vi "Hold to Roof_1 port_Save Sweep Data to csv.vi"(0 "Test Information":T2={"Exp Name"="Cold Switching", "Lot"="0233A", "Wafer"="15", "Die Type"="L22", "Die X "="6", "Die Y"="8", "Exp"="1", "Die X_Y"="8"}, 1 "Filepath":path, 2 "Selected Exp Settings":T5={"Floor_Sweep_Stop_V"=36.0, "Resistance Threshold"=1.0, "Floor_Sweep_Start_V"=36.0, "Floor_Sweep_Step_V"=1.0, "Roof_Sweep_Stop_V"=36.0, "Roof_Sweep_Start_V"=36.0, "Roof_Sweep_Step_V"=1.0, "Experiment Name"="", "Meas_Type"=[0, 2, 4]}, 4 "Meas Type":string="QuickView_", 5 "Date Cluster":T3, 7 "Time":dbl[](array[numeric]), 9 "ks5080A_Meaurements":T4, 12 "PreTest Capacitance":dbl[](array[numeric]), 14 "PostTest Capacitance":dbl[](array[numeric])) -> ()   [LabVIEW 2013]
uses:
  Controls/Date Control.ctl
  Controls/Test Information.ctl
  Controls/ks5080A_Measurements.ctl
  Controls/Individual User Inputs_MultiTest.ctl
  Controls/Test Selection.ctl
  <vilib>/Utility/file.llb/Write To Spreadsheet File (string).vi
panel:
  in  "Tab Control":T1(tab)
  # "Calculation Settings"
  # "Test Settings"
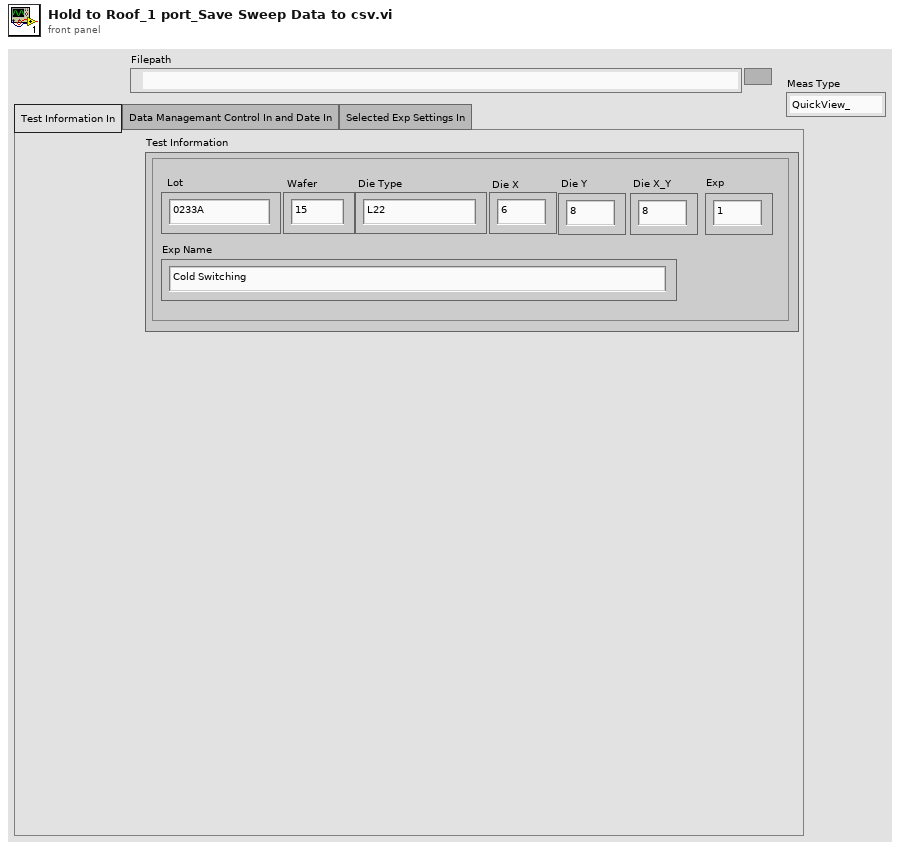
[diagram p1: front panel]
types:
  T1 = enum32{"Test Information In", "Data Managemant Control In and Date In", "Selected Exp Settings In"}
  T2 = typedef "Test Information.ctl" = cluster{"Exp Name":string, "Lot":string, "Wafer":string, "Die Type":string, "Die X ":string, "Die Y":string, "Exp":string, "Die X_Y":string}
  T3 = typedef "Date Control.ctl" = cluster{"Date":string, "Start Time":string, "Stop Time":string}
  T4 = typedef "ks5080A_Measurements.ctl" = cluster{"Bias_Sweep_Setting":dbl[], "Bias_voltage measurements":dbl[], "Bias_current measurements":dbl[], "P1_Capacitance":dbl[], "P2_Capacitance":dbl[], "DMM_Measurement_V":dbl[], "Contact_Source Current measurements":dbl[], "Contact_Sink Current measurements":dbl[], "Calculated_Resistance":dbl[], "P3_Capacitance":dbl[], "Port 1_S_parm":string[], "Port 2_S_parm":string[], "Port 3_S_parm":string[]}
  T5 = typedef "Individual User Inputs_MultiTest.ctl" = cluster{"Floor_Sweep_Stop_V":dbl, "Resistance Threshold":dbl, "Floor_Sweep_Start_V":dbl, "Floor_Sweep_Step_V":dbl, "Roof_Sweep_Stop_V":dbl, "Roof_Sweep_Start_V":dbl, "Roof_Sweep_Step_V":dbl, "Experiment Name":string, "Meas_Type":T6}
  T6 = typedef "Test Selection.ctl" = i32[]
  T7 = enum16{"open", "replace", "create", "open or create", "replace or create", "replace or create with confirmation"}
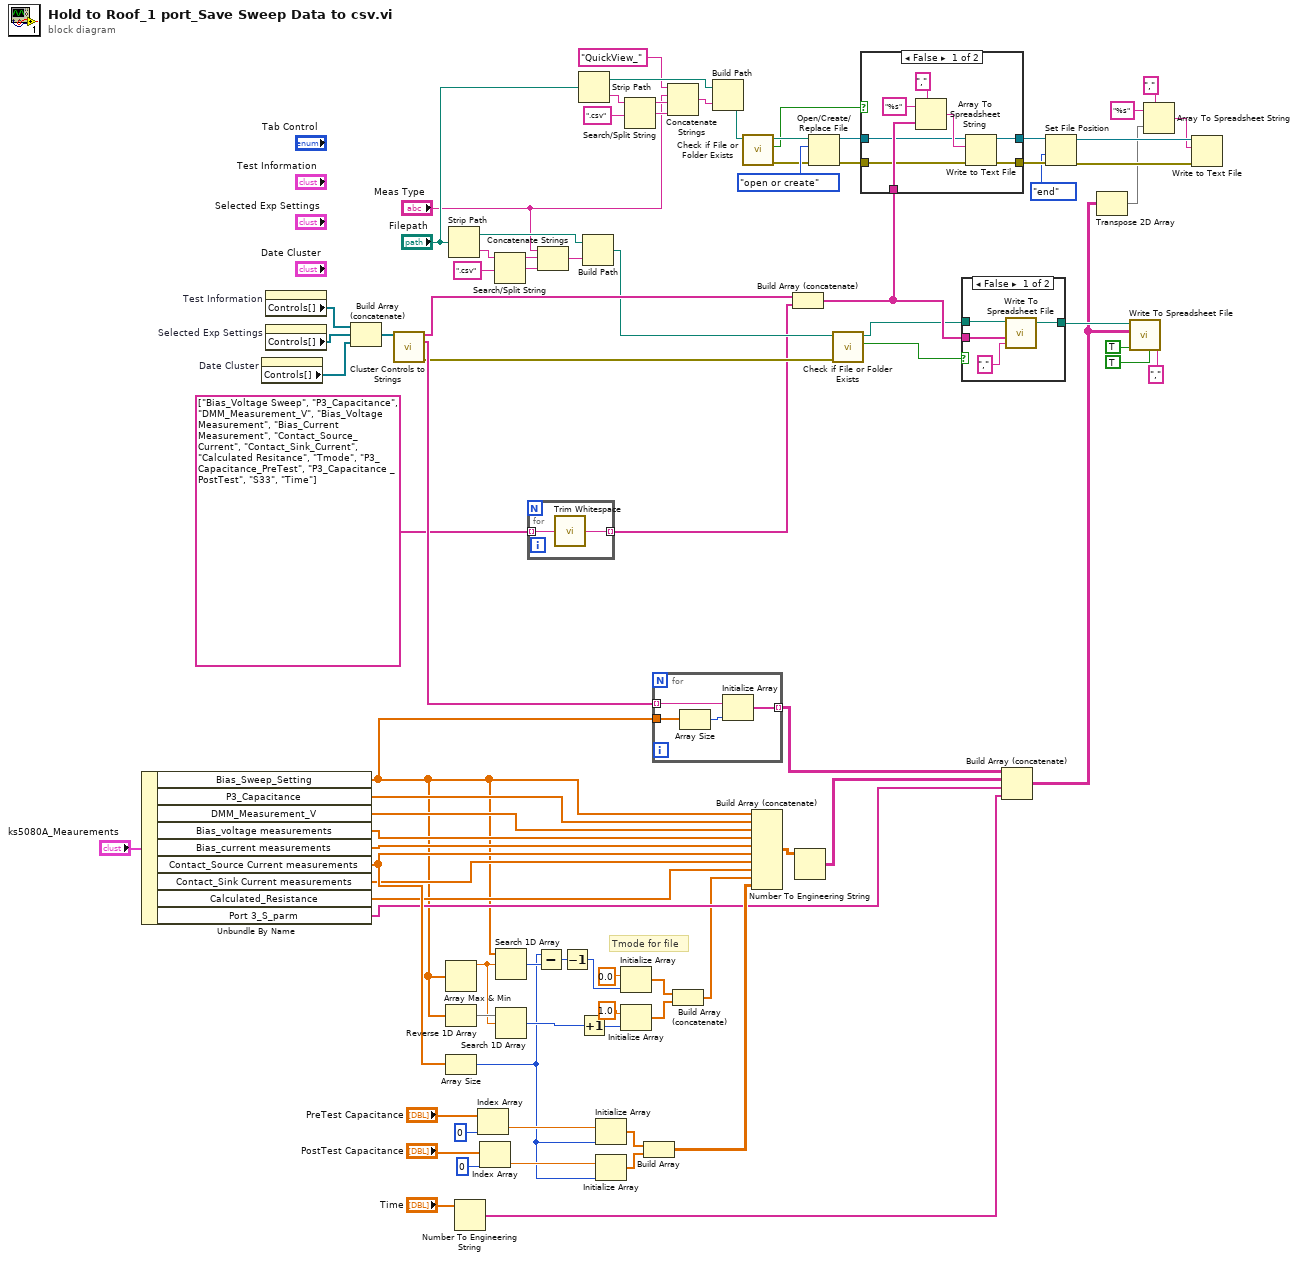
[diagram p0: block diagram]
diagram:
  # "Tmode for file"
  n1 = Unbundle By Name("ks5080A_Meaurements") -> ("Bias_Sweep_Setting"=w12:dbl[], "P3_Capacitance"=w83:dbl[], "DMM_Measurement_V"=w82:dbl[], "Bias_voltage measurements"=w81:dbl[], "Bias_current measurements"=w80:dbl[], "Contact_Source Current measurements"=w79:dbl[], "Contact_Sink Current measurements"=w48:dbl[], "Calculated_Resistance"=w47:dbl[], "Port 3_S_parm"=w30:string[])
  n2 = property on="Date Cluster" class="Clust (strict)"() -> ("Controls[]"=w1:refnum<vi>[])  [unwired: 2 in, 2 out]
  n3 = property on="Test Information" class="Clust (strict)"() -> ("Controls[]"=w86:refnum<vi>[])  [unwired: 2 in, 2 out]
  n4 = property on="Selected Exp Settings" class="Clust (strict)"() -> ("Controls[]"=w10:refnum<vi>[])  [unwired: 2 in, 2 out]
  n5 = Build Array (concatenate)(w86, w10, w1) -> (w85:refnum<vi>[])
  n6 = call "Cluster Controls to Strings.vi"("Controls[]"=w85) -> ("Control Labels"=w71:string[], "Control Values"=w84:string[], "Error Out"=w70:errorcluster)  [unwired: 12 in]
  n7 = Array Max & Min(array=w12) -> (max value=w19:dbl)  [unwired: 3 out]
  n8 = Reverse 1D Array(array=w12) -> (reversed array=w20:dbl[])
  n9 = Array Size(array=w79) -> (size(s)=w13:i32)
  n10 = Strip Path(path="Filepath") -> (stripped path=w33:path, name=w36:string)
  n11 = Number To Engineering String(4:"Time") -> (0:w8:string[])  [unwired: 3 in]
  n12 = Index Array(array="PreTest Capacitance", index=0) -> (element=w44:dbl)
  n13 = Index Array(array="PostTest Capacitance", index=0) -> (element=w43:dbl)
  n14 = Search/Split String(string=w36, search string/char (-)=".csv" ("search string")) -> (substring before match=w31:string, match + rest of string=w34:string)  [unwired: 1 in, 1 out]
  n15 = Search 1D Array(1D array=w12, element=w19) -> (index of element=w18:i32)  [unwired: 1 in]
  n16 = Search 1D Array(1D array=w20, element=w19) -> (index of element=w15:i32)  [unwired: 1 in]
  n17 = for {
    tunnel: string[] ["Bias_Voltage Sweep", "P3_Capacitance", "DMM_Measurement_V", "Bias_Voltage Measurement", "Bias_Current Measurement", "Contact_Source_Current", "Contact_Sink_Current", "Calculated Resitance", "Tmode", "P3_Capacitance_PreTest", "P3_Capacitance _PostTest", "S33", "Time"] -> [w88] mode=indexing
    tunnel: [w87] -> w2 mode=indexing
    n18 = call <vilib>:"Trim Whitespace.vi"("string"=w88) -> ("trimmed string"=w87:string)  [unwired: 1 in]
  }
  n19 = Subtract(x=w13, y=w18) -> (x-y=w17:i32)
  n20 = Concatenate Strings("Meas Type", w31, w34) -> (w32:string)
  n21 = Decrement(x=w17) -> (x-1=w16:i32)
  n22 = Strip Path(path="Filepath") -> (stripped path=w65:path, name=w68:string)
  n23 = Increment(x=w15) -> (x+1=w14:i32)
  n24 = Build Path(base path=w33, name or relative path=w32) -> (appended path=w7:path)
  n25 = Initialize Array(w44, w13) -> (w42:dbl[])
  n26 = Initialize Array(w43, w13) -> (w41:dbl[])
  n27 = Initialize Array(0.0, w16) -> (w24:dbl[])
  n28 = Initialize Array(1.0, w14) -> (w21:dbl[])
  n29 = Search/Split String(string=w68, search string/char (-)=".csv" ("search string")) -> (substring before match=w63:string, match + rest of string=w66:string)  [unwired: 1 in, 1 out]
  n30 = Build Array(w42, w41) -> (w40:dbl[][])
  n31 = for {
    tunnel: w12 -> [w92]
    tunnel: w84 -> [w91] mode=indexing
    tunnel: [w89] -> w74 mode=indexing
    n32 = Array Size(array=w92) -> (size(s)=w90:i32)
    n33 = Initialize Array(w91, w90) -> (w89:string[])
  }
  n34 = Concatenate Strings("QuickView_" ("search string"), "Meas Type", w63, w66) -> (w64:string)
  n35 = Build Array (concatenate)(w24, w21) -> (w11:dbl[])
  n36 = Build Path(base path=w65, name or relative path=w64) -> (appended path=w28:path)
  n37 = call <vilib>:"Check if File or Folder Exists.vi"("path"=w28) -> ("error out"=w29:errorcluster, "file or folder exists?"=w26:bool, "dup path"=w27:path)  [unwired: 8 in]
  n38 = Build Array (concatenate)(w12, w83, w82, w81, w80, w79, w48, w47, w11, w40) -> (w72:dbl[][])
  n39 = Build Array (concatenate)(w71, w2) -> (w61:string[])
  n40 = Number To Engineering String(4:w72) -> (0:w73:string[][])  [unwired: 3 in]
  n41 = Open/Create/Replace File(file path (use dialog)=w27, error in=w29, operation (0:open)=T7."open or create") -> (refnum out=w60:refnum<file>, error out=w59:errorcluster)  [unwired: 3 in, 1 out]
  n42 = call <vilib>:"Check if File or Folder Exists.vi"("error in (no error)"=w70, "path"=w7) -> ("file or folder exists?"=w62:bool, "dup path"=w25:path)  [unwired: 7 in, 1 out]
  n43 = case shown="False" w26 {
    tunnel: w61 -> [w98 _]
    tunnel: w60 -> [w96 w102]
    tunnel: w59 -> [w95 w101]
    tunnel: [w94 w101] -> w57
    tunnel: [w93 w102] -> w58
    frame False {
      n44 = Array To Spreadsheet String(delimiter (Tab)="," ("delimiter (\\t)"), array=w98, 3:"%s" ("format string")) -> (spreadsheet string=w97:string)
      n45 = Write to Text File(file (use dialog)=w96, text=w97, error in=w95) -> (refnum out=w93:refnum<file>, error out=w94:errorcluster)  [unwired: 1 in, 1 out]
    }
    frame True {
    }
  }
  n46 = case shown="False" w62 {
    tunnel: w25 -> [w106 w107]
    tunnel: w61 -> [w105 _]
    tunnel: [w103 w107] -> w78
    frame False {
      n47 = call-poly <vilib>:"Write To Spreadsheet File.vi"("delimiter (\\t)"="," ("delimiter (\\t)"), "1D data"=w105, "file path (dialog if empty)"=w106) -> ("new file path (Not A Path if cancelled)"=w103:path)  [unwired: 5 in]
    }
    frame True {
    }
  }
  n48 = Build Array (concatenate)(w74, w73, w30, w8) -> (w50:string[][])
  n49 = Set File Position(refnum=w58, from (0:start)=enum16{"start", "end", "current"}."end", error in=w57) -> (refnum out=w52:refnum<file>, error out=w53:errorcluster)  [unwired: 1 in]
  n50 = Transpose 2D Array(2D array=w50) -> (transposed array=w49:string[][])
  n51 = call-poly <vilib>:"Write To Spreadsheet File.vi"("delimiter (\\t)"="," ("delimiter (\\t)"), "transpose? (no:F)"=TRUE, "append to file? (new file:F)"=TRUE, "2D data"=w50, "file path (dialog if empty)"=w78) -> ()  [unwired: 3 in, 1 out]
  n52 = Array To Spreadsheet String(delimiter (Tab)="," ("delimiter (\\t)"), array=w49, 3:"%s" ("format string")) -> (spreadsheet string=w51:string)
  n53 = Write to Text File(file (use dialog)=w52, text=w51, error in=w53) -> ()  [unwired: 1 in, 3 out]
